vi "convertRawTimestamp.vi"(8 "error in (no error)":errorcluster, 10 "RawTimestamp":u64, 11 "Timestamp in":refnum<class "Timestamp.lvclass">) -> (0 "error out":errorcluster, 2 "Timestamp":dbl format="%#.6g", 3 "Timestamp out":refnum<class "Timestamp.lvclass">)   [LabVIEW 2016, in "RTTimestamp.lvlib" / "Timestamp.lvclass"]
uses:
  Timestamp.lvclass
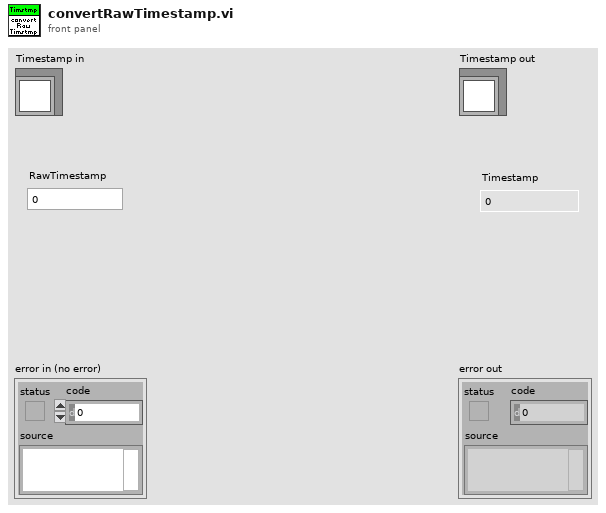
[diagram p1: front panel]
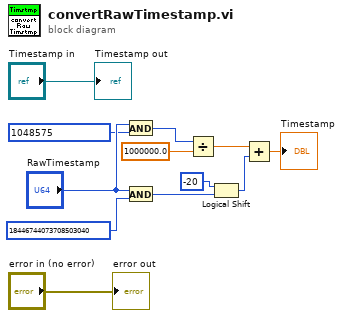
[diagram p0: block diagram]
diagram:
  n1 = And(x="RawTimestamp", y=u64 1048575) -> (x .and. y?=w7:u64)
  n2 = And(x="RawTimestamp", y=u64 18446744073708503040) -> (x .and. y?=w9:u64)
  n3 = Divide(x=w7, y=1000000.0) -> (x/y=w5:dbl)
  n4 = Logical Shift(y=i16 -20, x=w9) -> (x << y=w4:u64)
  n5 = Add(x=w5, y=w4) -> (x+y=→"Timestamp":dbl)
  "error out" <- "error in (no error)"
  "Timestamp out" <- "Timestamp in"
